vi "midi_ToMinSec.vi"(1 "seconds":dbl) -> (0 "min:sec":string)   [LabVIEW 2013]
doc: "Convert a numerical value (in seconds) to a string of the form min:sec."
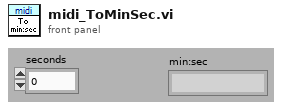
[diagram p1: front panel]
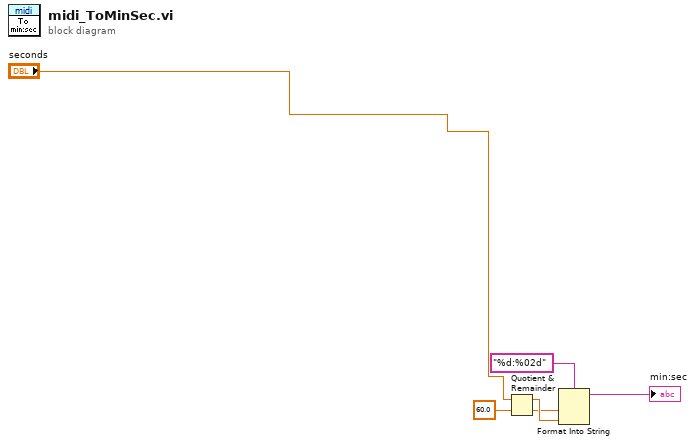
[diagram p0: block diagram]
diagram:
  n1 = Quotient & Remainder(x="seconds", y=60.0) -> (x-y*floor(x/y)=w5:dbl, floor(x/y)=w4:dbl)
  n2 = Format Into String(format string="%d:%02d", w4, w5) -> (resulting string=→"min:sec":string)  [unwired: 2 in, 1 out]
